vi "Add card dialog.vi"(8 "error in (no error)":errorcluster, 10 "Card Type in":string, 11 "Node Ptr":u64 format="%.0x") -> (0 "error out":errorcluster, 1 "Card position out":T1, 2 "Name out":string, 3 "Node Ptr out":u64 format="%.0x", 4 "Cancelled?":bool)   [LabVIEW 2013, in "SLSC configuration System Explorer.lvlib"]
uses:
  SLSC configuration System Explorer.lvlib
  Shared/Card Postion.ctl
  Shared/Constants.vi
  <vilib>/NI Veristand/Custom Device API/Custom Device API.lvlib
  Shared/SLSC configuration Shared.lvlib
panel:
  in  "Card position":T1 caption="Enter slot number"
  in  "Name":string
  in  "Cancel":bool
  in  "Add":bool
  out "Card Type":string
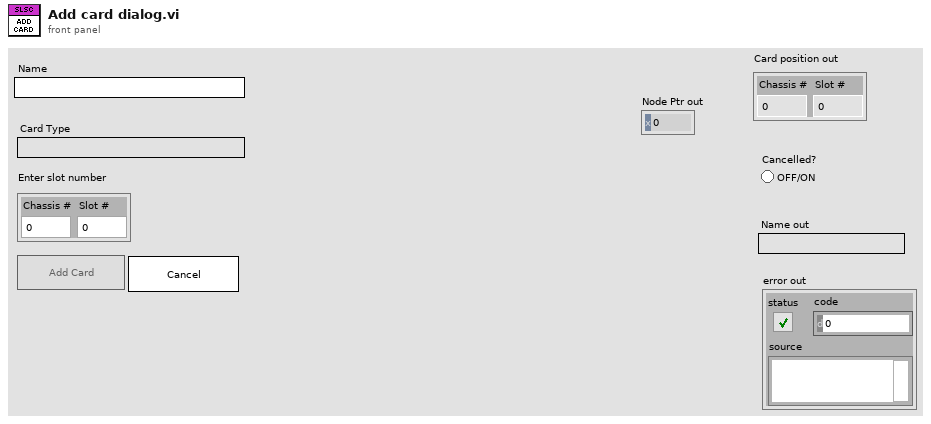
[diagram p1: front panel]
types:
  T1 = typedef "SLSC configuration Shared.lvlib/Card Postion.ctl" = cluster{"Chassis #":u8, "Slot #":u8}
  T2 = enum8{"Enabled", "Disabled", "Disabled and Grayed Out"}
  T3 = typedef "Custom Device API.lvlib/Custom Device Item Ref.ctl" = u64
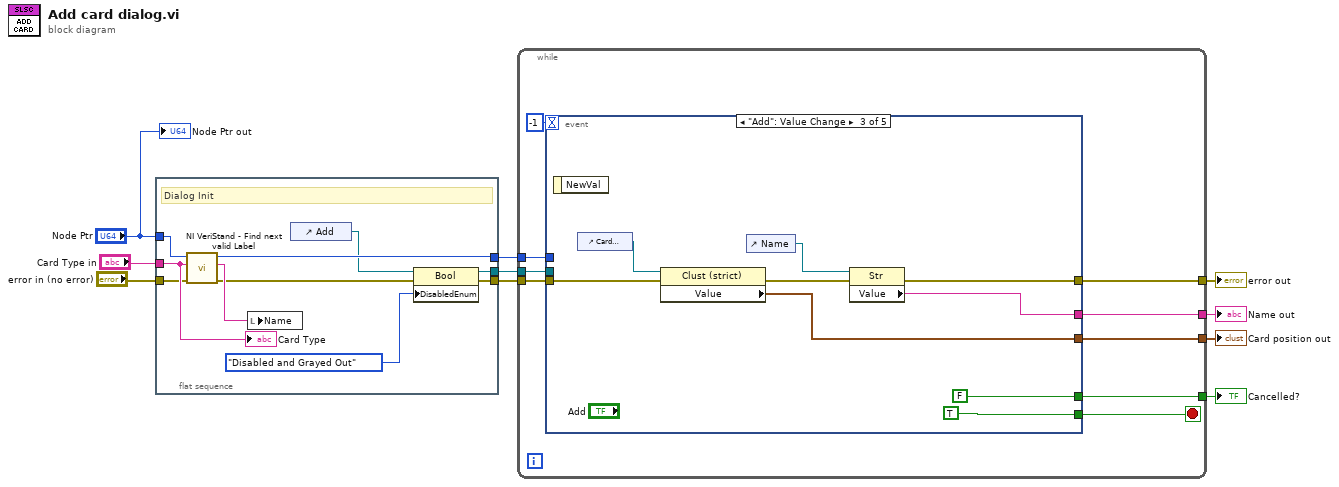
[diagram p0: block diagram]
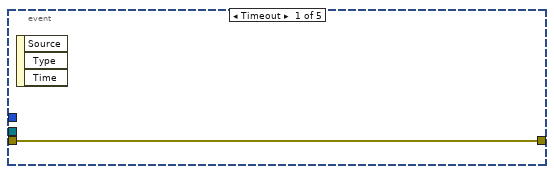
[diagram p2: hidden frame]
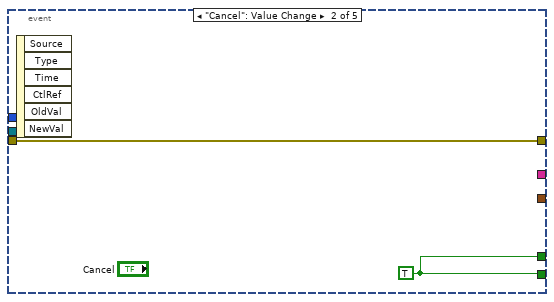
[diagram p3: hidden frame]
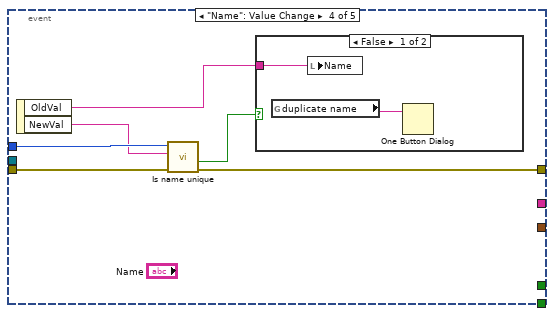
[diagram p4: hidden frame]
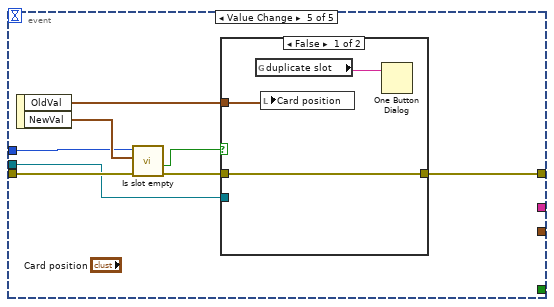
[diagram p6: hidden frame]
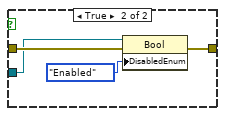
[diagram p7: hidden frame]
diagram:
  n1 = flat-sequence {
    tunnel: "Card Type in" -> [w20]
    tunnel: "error in (no error)" -> [w19]
    tunnel: "Node Ptr" -> [w12]
    tunnel: [w17] -> w7
    tunnel: [w15] -> w5
    tunnel: [w14] -> w4
    frame #0 {
      # "Dialog Init"
      n2 = call <vilib>:"NI VeriStand - Find next valid Label.vi"("error in (no error)"=w19, "Label"=w20, "Item Ref in"=w12) -> ("error out"=w16:errorcluster, "Label out"=w18:string, "Item Ref out"=w17:T3)  [unwired: 4 in, 2 out]
      n3 = local write "Name"(w18) -> ()
      n4 = control-ref of="Add"() -> (w11:refnum<vi>)
      n5 = property class="Bool"(reference=w11, error in=w16, "DisabledEnum"=T2."Disabled and Grayed Out" ("Disabled")) -> (reference out=w14:refnum<vi>, error out=w15:errorcluster)
      "Card Type" <- w20
    }
  }
  n6 = while {
    tunnel: w7 -> [w28]
    tunnel: w5 -> [w27]
    tunnel: [w26] -> w6
    tunnel: w4 -> [w25]
    tunnel: [w24] -> w3
    tunnel: [w22] -> w2
    tunnel: [w21] -> w1
    stop <- w29 stop-if-true
    n7 = event shown="[2] \"Add\": Value Change" {
      selector: _ -> [_ _ _ _ _]
      dyn-events: _ -> [_ _ _ _ _]
      timeout: -1 -> [_ _ _ _ _]
      tunnel: [_ w32 TRUE ("Cancel") _ _] -> w29
      tunnel: w28 -> [_ _ _ w46 w50]
      tunnel: w27 -> [w30 w31 w39 w45 w57]
      tunnel: [_ w32 FALSE ("Cancel") _ _] -> w26
      tunnel: w25 -> [_ _ _ _ w53]
      tunnel: [w30 w31 w35 w42 w51] -> w24
      tunnel: [_ _ w34 _ _] -> w22
      tunnel: [_ _ w33 _ _] -> w21
      event Timeout {
        n8 = event-data() -> ()  [unwired: 1 in, 3 out]
      }
      event "Cancel": Value Change {
        w32 = TRUE ("Cancel")
        n9 = event-data() -> ()  [unwired: 1 in, 6 out]
      }
      event "Add": Value Change {
        n10 = event-data() -> ()  [unwired: 1 in, 1 out]
        n11 = control-ref of="Card position"() -> (w38:refnum<vi>)
        n12 = property class="Clust (strict)"(reference=w38, error in=w39) -> (error out=w37:errorcluster, "Value"=w33:T1)  [unwired: 1 out]
        n13 = control-ref of="Name"() -> (w36:refnum<vi>)
        n14 = property class="Str"(reference=w36, error in=w37) -> (error out=w35:errorcluster, "Value"=w34:string)  [unwired: 1 out]
      }
      event "Name": Value Change {
        n15 = event-data() -> ("OldVal"=w47:string, "NewVal"=w43:string)  [unwired: 1 in]
        n16 = call "Is name unique.vi"("error in (no error)"=w45, "Name"=w43, "Node Ptr"=w46) -> ("error out"=w42:errorcluster, "Is name unique?"=w44:bool)  [unwired: 6 in, 1 out]
        n17 = case shown="False" w44 {
          tunnel: w47 -> [w49 _]
          frame False {
            n18 = global read "Constants.vi" "duplicate name"() -> (w48:string)
            n19 = local write "Name"(w49) -> ()
            n20 = One Button Dialog(message=w48) -> ()  [unwired: 1 in, 1 out]
          }
          frame True {
          }
        }
      }
      event Value Change {
        n21 = event-data() -> ("OldVal"=w55:T1, "NewVal"=w56:T1)  [unwired: 1 in]
        n22 = call "Is slot empty.vi"("error in (no error)"=w57, "Card Position"=w56, "Node Ptr"=w50) -> ("error out"=w52:errorcluster, "Empty?"=w54:bool)  [unwired: 6 in, 1 out]
        n23 = case shown="False" w54 {
          tunnel: w55 -> [w60 _]
          tunnel: w53 -> [_ w63]
          tunnel: w52 -> [w58 w64]
          tunnel: [w58 w61] -> w51
          frame False {
            n24 = global read "Constants.vi" "duplicate slot"() -> (w59:string)
            n25 = local write "Card position"(w60) -> ()
            n26 = One Button Dialog(message=w59) -> ()  [unwired: 1 in, 1 out]
          }
          frame True {
            n27 = property class="Bool"(reference=w63, error in=w64, "DisabledEnum"=T2."Enabled" ("Disabled")) -> (error out=w61:errorcluster)  [unwired: 1 out]
          }
        }
      }
    }
  }
  "Cancelled?" <- w6
  "error out" <- w3
  "Name out" <- w2
  "Card position out" <- w1
  "Node Ptr out" <- "Node Ptr"
